vi "PKG_IMC_SetParamBit.vi"(5 "fifo":i32, 6 "axis":i32, 7 "val":i16, 9 "bit":i16, 10 "paramloc":i16, 11 "Handle":u32) -> (2 "function return":i32, 3 "Handle out":u32)   [LabVIEW 2018, in "IMC_Pkg4xxx.lvlib"]
doc: "PKG_IMC_SetParamBit(IMC_HANDLE Handle, short paramloc, short bit, short val, int axis, int fifo);"
uses:
  IMC_Pkg4xxx.lvlib
  IMC_Pkg4xxx.dll
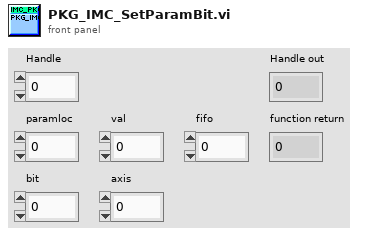
[diagram p1: front panel]
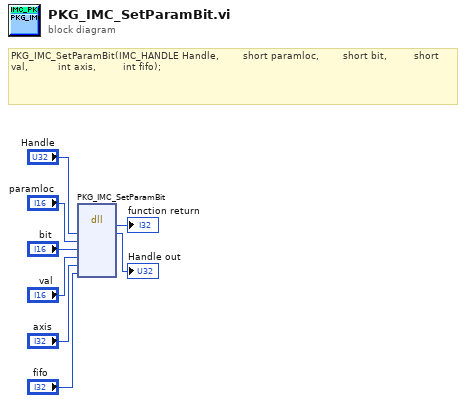
[diagram p0: block diagram]
diagram:
  # "PKG_IMC_SetParamBit(IMC_HANDLE Handle, \t\t\t\t\t\t\tshort paramloc, \t\t\t\t\t\t\tshort bit,\t\t\t\t\t\t\t\t\tshort val, \t\t\t\t\t\t\t\t\tint axis,\t\t\t\t\t\t\t\t\tint fifo);"
  n1 = dll-call lib="PTH2\\abs D做的项目航天测量驱动电机IMCAppincLabview32\nIMC_Pkg4xxx.*" fn="PKG_IMC_SetParamBit"("Handle"="Handle", "paramloc"="paramloc", "bit"="bit", "val"="val", "axis"="axis", "fifo"="fifo") -> (→"function return":i32, "Handle"=→"Handle out":u32)  [unwired: 8 in, 2 out]
